vi "FPGAMemoryInit_Palette_FXP.vi"() -> (0 "Init Data Out":fxp<+,8,8>[](array[numeric]) format="%08b")   [LabVIEW 2020]
uses:
  591418b3-9de5-4ac9-a68d-6cfd3e68fd08.vi
  57ced094-b5bd-4353-8baf-9025bca350fd.vi
panel:
  out "256 to 64 LUT":u8[](array[numeric])
  out "Palette":u32[](array[colorbox])
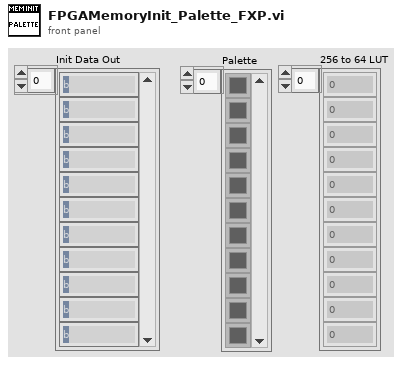
[diagram p1: front panel]
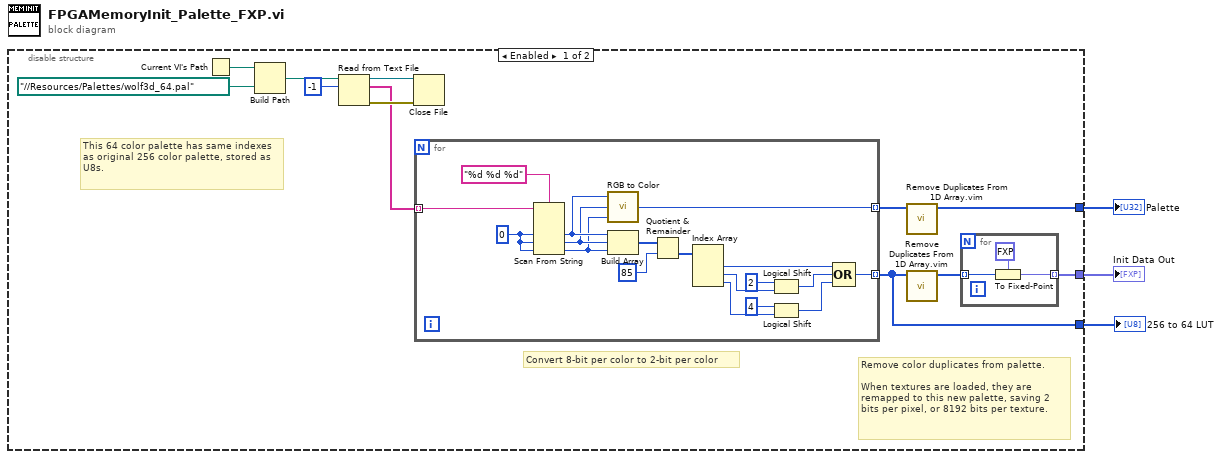
[diagram p0: block diagram]
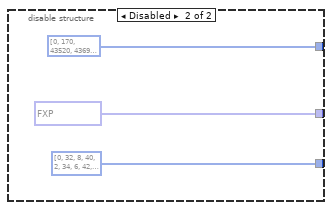
[diagram p2: hidden frame]
diagram:
  n1 = disable-structure shown="Enabled" {
    disable-tunnel: [w8 u32[] [0, 170, 43520, 43690, 11141120, 11141290, 11162880, 11184810, 5592405, 5592575, 5635925, 5636095, 16733525, 16733695, 16777045, 16777215, 16711680, 5570560, 16755370, 16755285, 16755200, 16733440, 16777130, 16776960, 11184640, 5592320, 11206485, 11206400, 5614080, 11206570, 65280, 21760, 11206655, 65535, 21845, 5614335, 43775, 21930, 11184895, 255, 85, 11141375, 5570730, 5570645, 16755455, 16711935, 11184725, 11162965, 5614250] ("Palette")] -> w3
    disable-tunnel: [w10 fxp<+,6,6>[] [0.0, 32.0, 8.0, 40.0, 2.0, 34.0, 6.0, 42.0, 21.0, 53.0, 29.0, 61.0, 23.0, 55.0, 31.0, 63.0, 3.0, 1.0, 43.0, 27.0, 11.0, 7.0, 47.0, 15.0, 10.0, 5.0, 30.0, 14.0, 9.0, 46.0, 12.0, 4.0, 62.0, 60.0, 20.0, 57.0, 56.0, 36.0, 58.0, 48.0, 16.0, 50.0, 33.0, 17.0, 59.0, 51.0, 26.0, 22.0, 41.0] ("Init Data Out")] -> w2
    disable-tunnel: [w7 u8[] [0, 32, 8, 40, 2, 34, 6, 42, 21, 53, 29, 61, 23, 55, 31, 63, 63, 63, 42, 42, 42, 42, 42, 42, 21, 21, 21, 21, 21, 21, 21, 0, 3, 3, 3, 2, 2, 2, 2, 2, 2, 2, 1, 1, 1, 1, 1, 1, 63, 43, 43, 23, 23, 23, 3, 3, 27, 27, 11, 7, 7, 6, 6, 6, 63, 47, 47, 31, 31, 31, 15, 15, 15, 10, 10, 10, 10, 5, 5, 5, 30, 30, 14, 14, 14, 10, 9, 9, 63, 46, 46, 30, 29, 29, 12, 12, 12, 12, 12, 8, 8, 8, 8, 8, 8, 8, 4, 4, 4, 4, 4, 4, 63, 62, 62, 61, 61, 61, 60, 60, 60, 40, 40, 40, 40, 20, 20, 20, 57, 57, 56, 56, 56, 36, 36, 36, 63, 58, 58, 57, 53, 53, 48, 48, 48, 48, 48, 32, 32, 32, 32, 32, 32, 32, 16, 16, 16, 16, 16, 16, 0, 31, 11, 11, 11, 11, 50, 50, 50, 34, 33, 33, 33, 17, 17, 16, 63, 59, 59, 55, 55, 55, 51, 51, 51, 34, 34, 34, 34, 17, 17, 17, 63, 47, 47, 43, 43, 43, 43, 43, 43, 27, 27, 27, 27, 27, 26, 22, 22, 22, 22, 22, 22, 22, 22, 22, 5, 5, 5, 5, 5, 5, 5, 0, 17, 20, 20, 0, 16, 1, 17, 17, 16, 0, 21, 21, 21, 21, 21, 63, 62, 62, 41, 41, 40, 40, 40, 40, 40, 40, 20, 20, 20, 20, 20, 34] ("Dupes")] -> w1
    frame Enabled {
      # "Remove color duplicates from palette.\n\nWhen textures are loaded, they are remapped to this new palette, saving 2 bits per pixel, or 8192 bits per texture."
      # "Convert 8-bit per color to 2-bit per color"
      # "This 64 color palette has same indexes as original 256 color palette, stored as U8s."
      n2 = Current VI's Path() -> (path=w6:path)
      n3 = Build Path(base path=w6, name or relative path=path "../../Resources/Palettes/wolf3d_64.pal") -> (appended path=w4:path)
      n4 = Read from Text File(file (use dialog)=w4, count=-1) -> (refnum out=w14:refnum<file>, text=w12:string[], error out=w13:errorcluster)  [unwired: 2 in, 1 out]
      n5 = Close File(refnum=w14, error in=w13) -> ()  [unwired: 2 out]
      n6 = for {
        tunnel: w12 -> [w35] mode=indexing
        tunnel: [w23] -> w7 mode=indexing
        tunnel: [w19] -> w9 mode=indexing
        w34 = u8 0 ("default value 1")
        n7 = Scan From String(format string="%d %d %d", input string=w35, default 1=w34, default 2=w34, default 3=w34) -> (output 1=w22:u8, output 2=w21:u8, output 3=w20:u8)  [unwired: 2 in, 3 out]
        n8 = call <vilib>:"RGB to Color.vi"("B"=w20, "G"=w21, "R"=w22) -> ("Color"=w19:u32)
        n9 = Build Array(w22, w21, w20) -> (w32:u8[])
        n10 = Quotient & Remainder(x=w32, y=u8 85) -> (floor(x/y)=w31:u8[])  [unwired: 1 out]
        n11 = Index Array(array=w31) -> (element #1=w26:u8, element #2=w30:u8, element #3=w27:u8)  [unwired: 3 in]
        n12 = Logical Shift(y=i16 2, x=w30) -> (x << y=w25:u8)
        n13 = Logical Shift(y=i16 4, x=w27) -> (x << y=w24:u8)
        n14 = Compound Arithmetic op=OR(w26, w25, w24) -> (w23:u8)
      }
      n15 = call "Remove Duplicates From 1D Array.vim"("array"=w9) -> ("array with duplicates removed"=w8:u32[])  [unwired: 10 in]
      n16 = call "Remove Duplicates From 1D Array.vim"("array"=w7) -> ("array with duplicates removed"=w11:u8[])  [unwired: 10 in]
      n17 = for {
        tunnel: w11 -> [w18] mode=indexing
        tunnel: [w17] -> w10 mode=indexing
        n18 = To Fixed-Point(fixed-point type=fxp<+,6,6> 0.0, number=w18) -> (fixed-point=w17:fxp<+,6,6>)
      }
    }
    frame Disabled {
    }
  }
  "Init Data Out" <- w2
  "Palette" <- w3
  "256 to 64 LUT" <- w1
